vi "UIRefs Flow Measured.vi"(8 "error in (no error)":errorcluster, 11 "FC2901 in":refnum<class "FC2901.lvclass">) -> (0 "error out":errorcluster, 3 "FC2901 out":refnum<class "FC2901.lvclass">)   [LabVIEW 2021, in "FC2901.lvclass"]
uses:
  FC2901.lvclass
  FC2901.lvclass/FC2901.ctl
  <vilib>/Utility/miscctls.llb/LVOutOfRangeActionTypeDef.ctl
  <vilib>/Utility/miscctls.llb/LVForegroundBackgroundColorsTypeDef.ctl
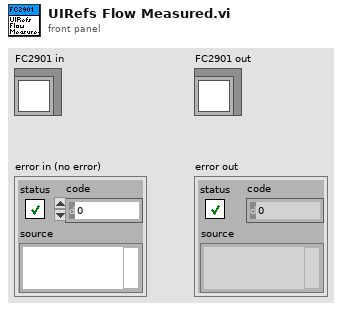
[diagram p1: front panel]
types:
  T1 = typedef "LVForegroundBackgroundColorsTypeDef.ctl" = cluster{"Foreground Color":u32, "Background Color":u32}
  T2 = typedef "LVOutOfRangeActionTypeDef.ctl" = cluster{"Out of Range Action Minimum":u8, "Out of Range Action Maximum":u8, "Out of Range Action Increment":u8}
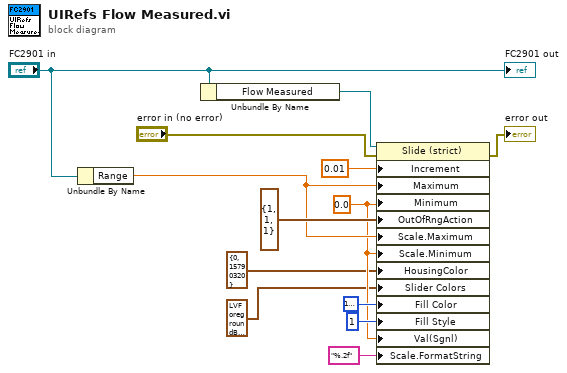
[diagram p0: block diagram]
diagram:
  w4 = 0.0 ("Data Entry Limits:Minimum")
  n1 = Unbundle By Name("FC2901 in") -> ("Range"=w5:dbl)
  n2 = Unbundle By Name("FC2901 in") -> ("Flow Measured"=w7:refnum<vi>)
  n3 = property class="Slide (strict)"(reference=w7, error in="error in (no error)", "Increment"=0.01 ("Data Entry Limits:Increment"), "Maximum"=w5, "Minimum"=w4, "OutOfRngAction"=T2 {"Out of Range Action Minimum"=1, "Out of Range Action Maximum"=1, "Out of Range Action Increment"=1} ("Response to Value Outside Limits"), "Scale.Maximum"=w5, "Scale.Minimum"=w4, "HousingColor"=T1 {"Foreground Color"=0, "Background Color"=15790320} ("Housing Colors"), "Slider Colors"=T1 {"Foreground Color"=16777216, "Background Color"=16777216}, "Fill Color"=u32 16777216, "Fill Style"=1, "Val(Sgnl)"=w4, "Scale.FormatString"="%.2f" ("Scale.Format String")) -> (error out=→"error out":errorcluster)  [unwired: 1 out]
  "FC2901 out" <- "FC2901 in"
